vi "Generate Test Data.vi"(11 "Single_Array in":refnum<class "Single_Array.lvclass">) -> (3 "Single_Array out":refnum<class "Single_Array.lvclass">)   [LabVIEW 2014, in "Base Data Class.lvlib" / "Single_Array.lvclass"]
uses:
  Single_Array.lvclass
  Single_Array.lvclass/Single_Array.ctl
  Data.lvclass
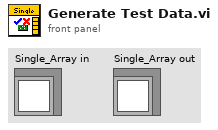
[diagram p1: front panel]
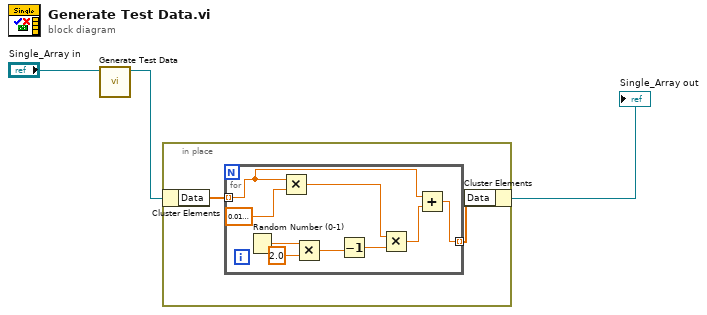
[diagram p0: block diagram]
diagram:
  n1 = call-parent "Generate Test Data.vi"("Data in"="Single_Array in") -> ("Data out"=w2:refnum<class "Single_Array.lvclass">)  [unwired: 10 in]
  n2 = in-place {
    n3 = in-place-cluster #1(w2) -> ("Data"=w4:sgl[])
    n4 = for {
      tunnel: [w6] -> w5 mode=indexing
      tunnel: w4 -> [w7] mode=indexing
      n5 = Random Number (0-1)() -> (number: 0 to 1=w13:dbl)
      n6 = Multiply(x=w7, y=sgl 0.02) -> (x*y=w9:sgl)
      n7 = Multiply(x=w13, y=2.0) -> (x*y=w11:dbl)
      n8 = Decrement(x=w11) -> (x-1=w10:dbl)
      n9 = Multiply(x=w9, y=w10) -> (x*y=w8:dbl)
      n10 = Add(x=w7, y=w8) -> (x+y=w6:dbl)
    }
    n11 = in-place-cluster #1("Data"=w5) -> (→"Single_Array out":refnum<class "Single_Array.lvclass">)
  }
